vi "Read.vi"(8 "error in":errorcluster) -> (0 "error out":errorcluster)   [LabVIEW 2018, in "ARINC.lvlib"]
doc: "This subVI enqueues the named action in to the communications queue along with the input data."
uses:
  ARINC.lvlib
  Private Controls/Module Data.ctl
  Private Controls/Module Action.ctl
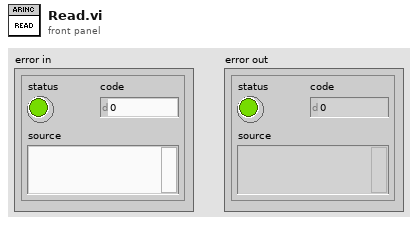
[diagram p1: front panel]
types:
  T1 = typedef "ARINC.lvlib/Module Data.ctl" = cluster{"Data":variant, "Action":T2}
  T2 = typedef "ARINC.lvlib/Module Action.ctl" = enum16{"Init", "Write(Tx)", "Read(Rx)", "Error"}
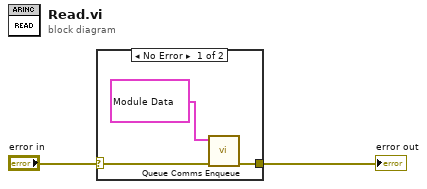
[diagram p0: block diagram]
diagram:
  n1 = case shown="No Error" "error in" {
    selector: "error in" -> [w4 w6]
    tunnel: [w5 w6] -> w2
    frame No Error {
      n2 = call "Queue Comms Enqueue.vi"("error in (no error)"=w4, "element"=T1 {"Data"=variant, "Action"=enum."Read(Rx)"}) -> ("error out"=w5:errorcluster)  [unwired: 9 in]
    }
    frame Error {
    }
  }
  "error out" <- w2
